vi "Target Data In.vi"(11 "writer name":refnum<k21>) -> (0 "Stop":bool)   [LabVIEW 2018]
uses:
  Host Messages.ctl
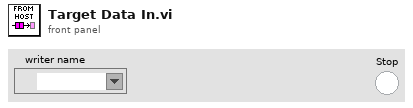
[diagram p1: front panel]
types:
  T1 = typedef "Host Messages.ctl" = enum16{"Stop", "Log Data", "Confirm File Name"}
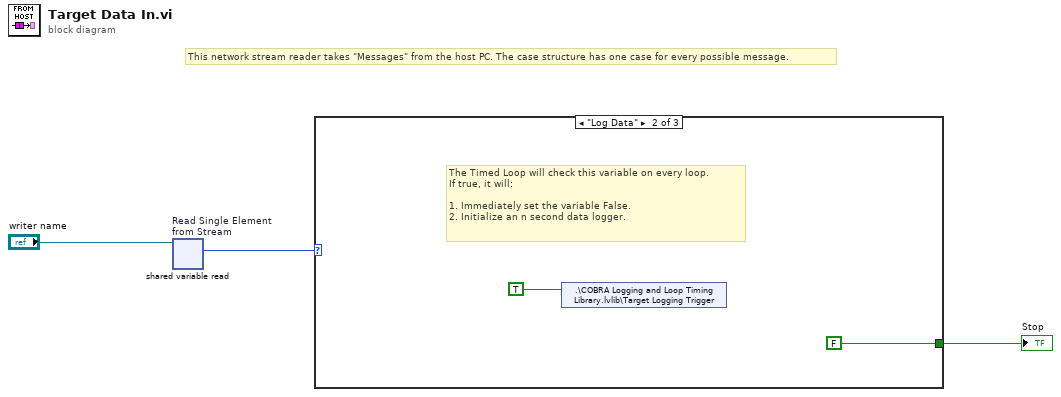
[diagram p0: block diagram]
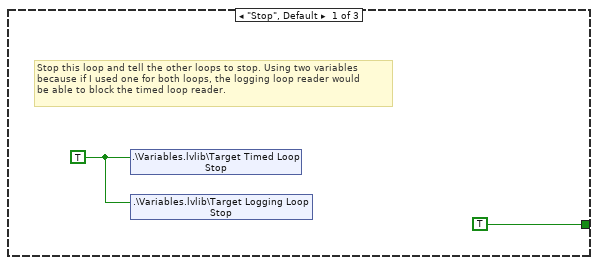
[diagram p2: hidden frame]
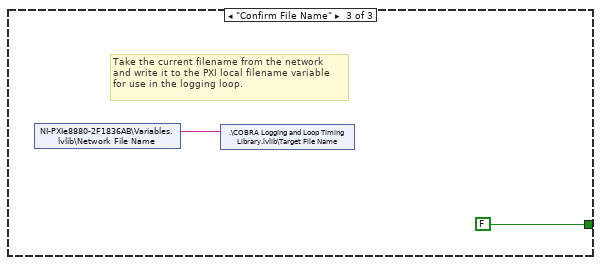
[diagram p3: hidden frame]
diagram:
  # "This network stream reader takes \"Messages\" from the host PC. The case structure has one case for every possible message."
  n1 = shared-variable-read "Read Single Element from Stream"("writer name") -> (w2:T1)  [unwired: 2 in, 3 out]
  n2 = case shown="\"Log Data\"" w2 {
    tunnel: [TRUE FALSE FALSE] -> w1
    frame "Stop", Default {
      w4 = TRUE ("PXI Timed Loop Stop")
      # "Stop this loop and tell the other loops to stop. Using two variables\nbecause if I used one for both loops, the logging loop reader would\nbe able to block the timed loop reader."
      n3 = shared-variable ".\\Variables.lvlib\\Target Timed Loop Stop"(w4) -> ()  [unwired: 1 in, 1 out]
      n4 = shared-variable ".\\Variables.lvlib\\Target Logging Loop Stop"(w4) -> ()  [unwired: 1 in, 1 out]
    }
    frame "Log Data" {
      # "The Timed Loop will check this variable on every loop.\nIf true, it will:\n\n1. Immediately set the variable False.\n2. Initialize an n second data logger."
      n5 = shared-variable ".\\COBRA Logging and Loop Timing Library.lvlib\\Target Logging Trigger"(TRUE ("PXI Log Trigger")) -> ()  [unwired: 1 in, 1 out]
    }
    frame "Confirm File Name" {
      # "Take the current filename from the network\nand write it to the PXI local filename variable\nfor use in the logging loop."
      n6 = shared-variable "NI-PXIe8880-2F1836AB\\Variables.lvlib\\Network File Name"() -> (w8:string)  [unwired: 1 in, 1 out]
      n7 = shared-variable ".\\COBRA Logging and Loop Timing Library.lvlib\\Target File Name"(w8) -> ()  [unwired: 1 in, 1 out]
    }
  }
  "Stop" <- w1
